vi "Aim.vi"(6 "Reset":bool, 10 "Angle":dbl, 11 "arm.lvclass":refnum<class "arm.lvclass">) -> (3 "arm.lvclass":refnum<class "arm.lvclass">)   [LabVIEW 2015, in "arm.lvclass"]
uses:
  arm.lvclass
  arm.lvclass/arm.ctl
  <vilib>/addons/control/pid/pid.llb/PID (DBL).vi
  <vilib>/addons/control/pid/NI_PID_pid.lvlib
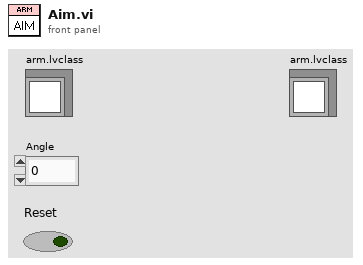
[diagram p1: front panel]
types:
  T1 = cluster{"proportional gain (Kc)":dbl, "integral time (Ti, min)":dbl, "derivative time (Td, min)":dbl}
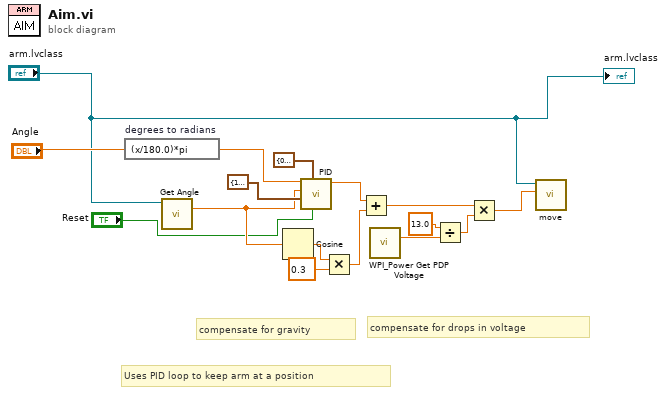
[diagram p0: block diagram]
diagram:
  # "Uses PID loop to keep arm at a position"
  # "compensate for drops in voltage"
  # "compensate for gravity"
  n1 = expression code="(x/180.0)*pi" "degrees to radians"("Angle") -> (w14:dbl)
  n2 = call "Get Angle.vi"("arm in"="arm.lvclass") -> ("Angle"=w4:dbl)  [unwired: 9 in, 1 out]
  n3 = Cosine(x=w4) -> (cos(x)=w12:dbl)
  n4 = call-poly <vilib>:"PID.vi"("reinitialize? (F)"="Reset", "output range"=cluster{"output high":dbl, "output low":dbl} {"output high"=0.7, "output low"=-0.7}, "PID gains"=T1 {"proportional gain (Kc)"=1.1, "integral time (Ti, min)"=0.008, "derivative time (Td, min)"=0.0001} ("PID arm gains"), "process variable"=w4, "setpoint"=w14) -> ("output"=w11:dbl)  [unwired: 5 in, 1 out]
  n5 = Multiply(x=w12, y=0.3) -> (x*y=w10:dbl)
  n6 = Add(x=w11, y=w10) -> (x+y=w7:dbl)
  n7 = call <vilib>:"WPI_Power Get PDP Voltage.vi"() -> ("voltage (V)"=w8:dbl)  [unwired: 14 in, 1 out]
  n8 = Divide(x=13.0, y=w8) -> (x/y=w6:dbl)
  n9 = Multiply(x=w7, y=w6) -> (x*y=w5:dbl)
  n10 = call "move.vi"("Speed"=w5, "arm.lvclass"="arm.lvclass") -> ()  [unwired: 9 in, 1 out]
  "arm.lvclass" <- "arm.lvclass"
